vi "读取外设配置.vi"(8 "error in (no error)":errorcluster, 11 "MB session in":refnum<class "MB_Master.lvclass">) -> (0 "error out":errorcluster, 2 "外设配置":T1 {"总氮x公式0" items=["0", "1"]; "光谱仪类型" items=["1型", "2型", "3型", "2型氙灯联控"]; "泵阀量" items=["9通"=9, "10通"=10, "12通"=12]; "泵类型" items=["1型", "2型", "sy04型+旋转阀"]}, 3 "MB session out":refnum<class "MB_Master.lvclass">)   [LabVIEW 2016, in "斯坦道氨氮.lvlib"]
uses:
  <vilib>/Plasmionique/MB Master/MB_Master/MB_Master.lvclass
  <vilib>/Plasmionique/MB Master/MB_Master_Serial/MB_Master_Serial.lvclass
  C:/Program Files (x86)/National Instruments/LabVIEW 2016/vi.lib/Plasmionique/MB Master/MB_Master/MB_Master.lvclass
  <vilib>/Plasmionique/MB Master/MB Master.lvlib
panel:
  in  "VISA Resource":refnum<visa-resource-name>
  in  "引用选择":enum16{"MB引用", "自建引用"}(ring)
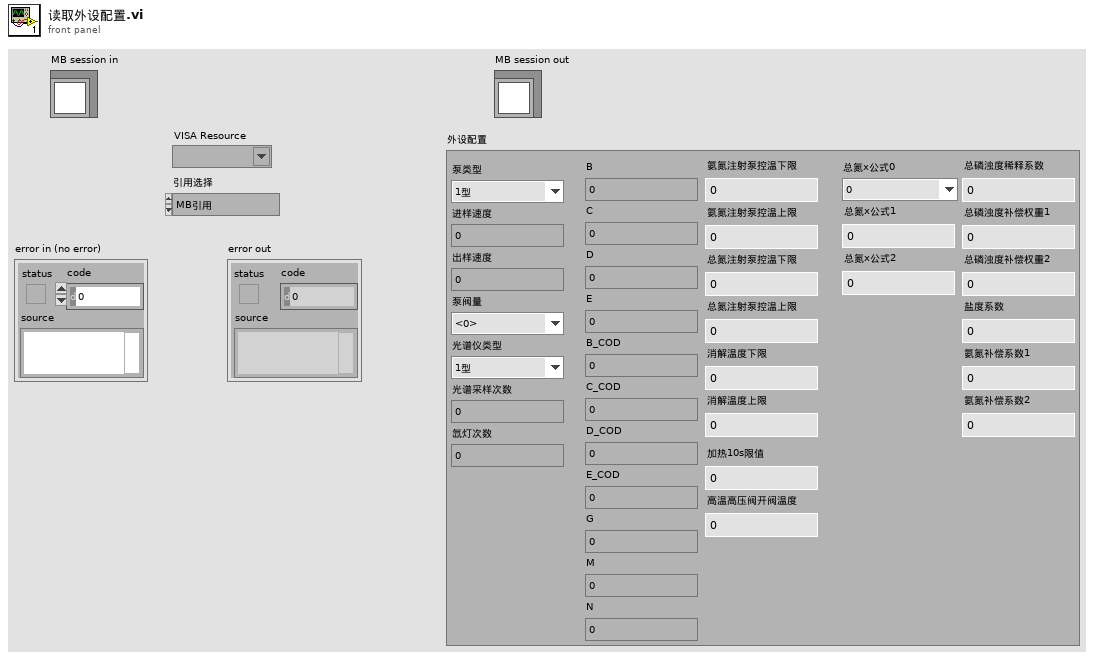
[diagram p1: front panel]
types:
  T1 = cluster{"泵类型":u8, "进样速度":u32, "出样速度":u32, "泵阀量":u8, "光谱仪类型":u8, "光谱采样次数":u8, "氙灯次数":u8, "B":u16, "C":u16, "D":u16, "E":u16, "B_COD":u16, "C_COD":u16, "D_COD":u16, "E_COD":u16, "G":u16, "M":u16, "N":u16, "氨氮注射泵控温下限":sgl, "氨氮注射泵控温上限":sgl, "总氮注射泵控温下限":sgl, "总氮注射泵控温上限":sgl, "消解温度下限":sgl, "消解温度上限":sgl, "加热10s限值":sgl, "高温高压阀开阀温度":sgl, "总氮x公式0":u8, "总氮x公式1":sgl, "总氮x公式2":sgl, "总磷浊度稀释系数":sgl, "总磷浊度补偿权重1":sgl, "总磷浊度补偿权重2":sgl, "盐度系数":sgl, "氨氮补偿系数1":sgl, "氨氮补偿系数2":sgl}
  T2 = cluster{"baud rate (bps)":u32, "stop bits":u16, "parity":u16, "flow control":u16, "timeout":u32, "retries":i32}
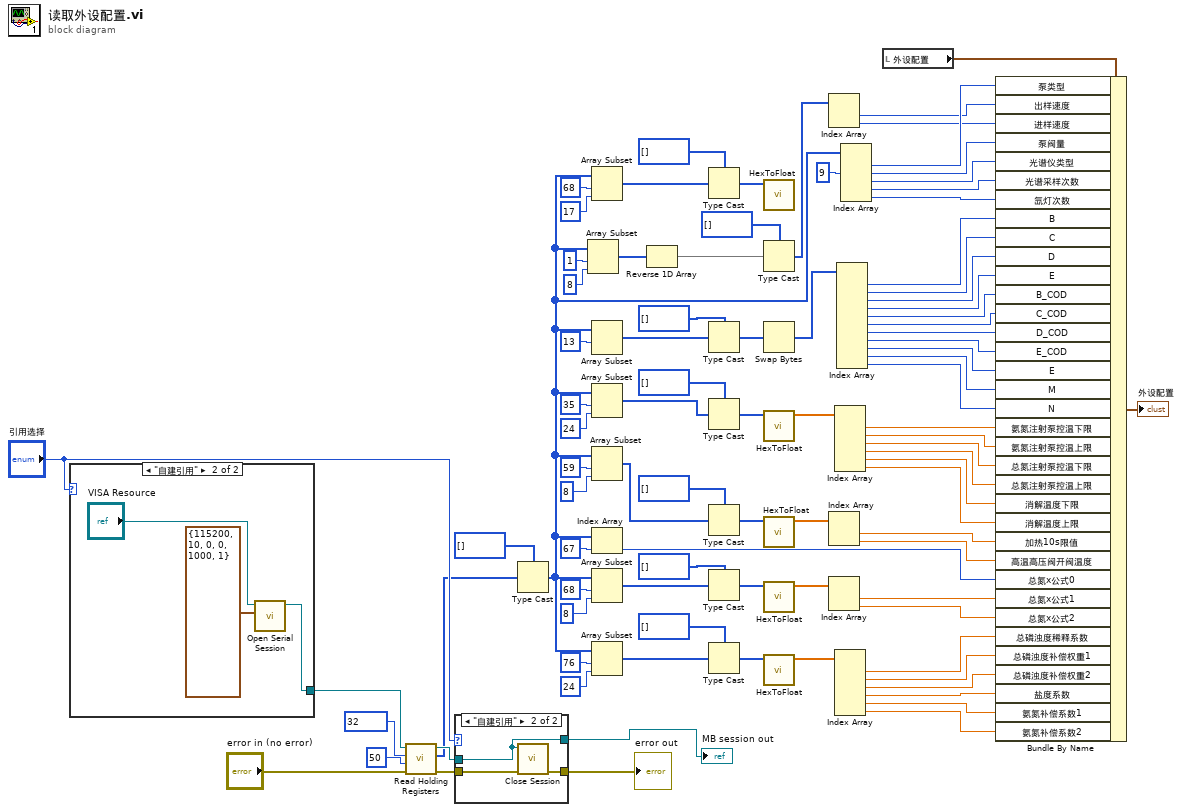
[diagram p0: block diagram]
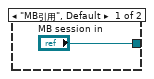
[diagram p3: hidden frame]
diagram:
  n1 = case shown="\"自建引用\"" "引用选择" {
    tunnel: ["MB session in" w95] -> w73
    frame "MB引用", Default {
    }
    frame "自建引用" {
      n2 = call <vilib>:"Open Serial Session.vi"("Serial Config"=T2 {"baud rate (bps)"=115200, "stop bits"=10, "parity"=0, "flow control"=0, "timeout"=1000, "retries"=1}, "VISA Resource"="VISA Resource") -> ("MB_Serial session"=w95:refnum<class "MB_Master_Serial.lvclass">)  [unwired: 8 in, 1 out]
    }
  }
  n3 = call <vilib>:"Read Holding Registers.vi"("error in (no error)"="error in (no error)", "quantity"=u16 50, "starting address"=u16 32, "MB session in"=w73) -> ("error out"=w69:errorcluster, "Registers"=w1:u16[], "MB session out"=w72:refnum<class "MB_Master.lvclass">)  [unwired: 5 in]
  n4 = case shown="\"自建引用\"" "引用选择" {
    tunnel: w72 -> [w96 w98]
    tunnel: w69 -> [w97 w100]
    tunnel: [w97 w99] -> w68
    tunnel: [w96 w98] -> w67
    frame "MB引用", Default {
    }
    frame "自建引用" {
      n5 = call-dynamic "Close Session.vi"("error in (no error)"=w100, "MB session in"=w98) -> ("error out"=w99:errorcluster)  [unwired: 9 in]
    }
  }
  "MB session out" <- w67
  "error out" <- w68
  n6 = Type Cast(type=u8[] [], x=w1) -> (*(type *) &x=w4:u8[])
  n7 = Array Subset(array=w4, index=1 ("索引"), length=8 ("长度")) -> (w82:u8[])
  n8 = Array Subset(array=w4, index=68 ("索引"), length=17 ("长度")) -> (w39:u8[])
  n9 = Array Subset(array=w4, index=13 ("索引")) -> (w34:u8[])  [unwired: 1 in]
  n10 = Array Subset(array=w4, index=35 ("索引"), length=24 ("长度")) -> (w57:u8[])
  n11 = Array Subset(array=w4, index=59 ("索引"), length=8 ("长度")) -> (w16:u8[])
  n12 = Index Array(array=w4, index=67 ("索引")) -> (element=w11:u8)
  n13 = Array Subset(array=w4, index=68 ("索引"), length=8 ("长度")) -> (w9:u8[])
  n14 = Array Subset(array=w4, index=76 ("索引"), length=24 ("长度")) -> (w50:u8[])
  n15 = Reverse 1D Array(array=w82) -> (reversed array=w81:u8[])
  n16 = Type Cast(type=u16[] [], x=w39) -> (*(type *) &x=w40:u16[])
  n17 = Type Cast(type=u16[] [], x=w34) -> (*(type *) &x=w33:u16[])
  n18 = Type Cast(type=u16[] [], x=w57) -> (*(type *) &x=w55:u16[])
  n19 = Type Cast(type=u16[] [], x=w16) -> (*(type *) &x=w17:u16[])
  n20 = Type Cast(type=u16[] [], x=w9) -> (*(type *) &x=w8:u16[])
  n21 = Type Cast(type=u16[] [], x=w50) -> (*(type *) &x=w52:u16[])
  n22 = call "HexToFloat.vi"("数组"=w40) -> ()  [unwired: 10 in, 1 out]
  n23 = Type Cast(type=u32[] [], x=w81) -> (*(type *) &x=w79:u32[])
  n24 = Swap Bytes(anything=w33) -> (byte swapped=w32:u16[])
  n25 = call "HexToFloat.vi"("数组"=w55) -> ("FLOAT"=w64:sgl[])  [unwired: 10 in]
  n26 = call "HexToFloat.vi"("数组"=w17) -> ("FLOAT"=w15:sgl[])  [unwired: 10 in]
  n27 = call "HexToFloat.vi"("数组"=w8) -> ("FLOAT"=w10:sgl[])  [unwired: 10 in]
  n28 = call "HexToFloat.vi"("数组"=w52) -> ("FLOAT"=w49:sgl[])  [unwired: 10 in]
  n29 = Index Array(array=w79) -> (element #1=w78:u32, element #2=w77:u32)  [unwired: 2 in]
  n30 = Index Array(array=w15) -> (element #1=w14:sgl, element #2=w13:sgl)  [unwired: 2 in]
  n31 = Index Array(array=w10) -> (element #1=w3:sgl, element #2=w2:sgl)  [unwired: 2 in]
  n32 = Index Array(array=w64) -> (element #1=w63:sgl, element #2=w62:sgl, element #3=w61:sgl, element #4=w60:sgl, element #5=w59:sgl, element #6=w58:sgl)  [unwired: 6 in]
  n33 = Index Array(array=w49) -> (element #1=w48:sgl, element #2=w47:sgl, element #3=w46:sgl, element #4=w45:sgl, element #5=w44:sgl, element #6=w43:sgl)  [unwired: 6 in]
  n34 = Index Array(array=w32) -> (element #1=w31:u16, element #2=w30:u16, element #3=w29:u16, element #4=w28:u16, element #5=w27:u16, element #6=w26:u16, element #7=w25:u16, element #8=w24:u16, element #9=w23:u16, element #10=w22:u16, element #11=w21:u16)  [unwired: 11 in]
  n35 = Index Array(array=w4, index #2=9 ("索引")) -> (element #1=w85:u8, element #2=w75:u8, element #3=w74:u8, element #4=w71:u8, element #5=w37:u8)  [unwired: 4 in]
  n36 = local read "外设配置"() -> (w87:T1)
  n37 = Bundle By Name(cluster=w87, "泵类型"=w85, "出样速度"=w78, "进样速度"=w77, "泵阀量"=w75, "光谱仪类型"=w74, "光谱采样次数"=w71, "氙灯次数"=w37, "B"=w31, "C"=w30, "D"=w29, "E"=w28, "B_COD"=w27, "C_COD"=w26, "D_COD"=w25, "E_COD"=w24, "E"=w23, "M"=w22, "N"=w21, "氨氮注射泵控温下限"=w63, "氨氮注射泵控温上限"=w62, "总氮注射泵控温下限"=w61, "总氮注射泵控温上限"=w60, "消解温度下限"=w59, "消解温度上限"=w58, "加热10s限值"=w14, "高温高压阀开阀温度"=w13, "总氮x公式0"=w11, "总氮x公式1"=w3, "总氮x公式2"=w2, "总磷浊度稀释系数"=w48, "总磷浊度补偿权重1"=w47, "总磷浊度补偿权重2"=w46, "盐度系数"=w45, "氨氮补偿系数1"=w44, "氨氮补偿系数2"=w43) -> (→"外设配置":T1)
